vi "XPath String Sub-Parser_Tran.vi"(8 "error in (no error)":errorcluster, 10 "XPath expression":string, 11 "XML String":string) -> (0 "error out":errorcluster, 2 "Array of Results":string[](array[string]), 3 "XML String out":string)   [LabVIEW 2019]
doc: "Use an XPath expression to search an XML string. An array containing all instances matching the search criteria will be returned.\n\nFor more information on XPath: http://www.w3schools.com/xpath/xpath_intro.asp"
uses:
  <vilib>/xml/Close Reference(Node).vi
  <vilib>/xml/NI_XML.lvlib
  <resource>/objmgr/DOMUserDefRef.rc
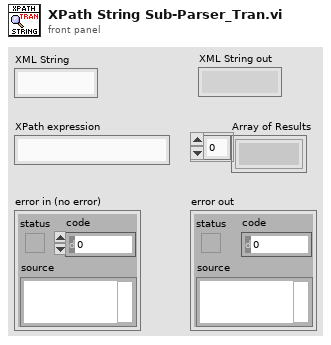
[diagram p1: front panel]
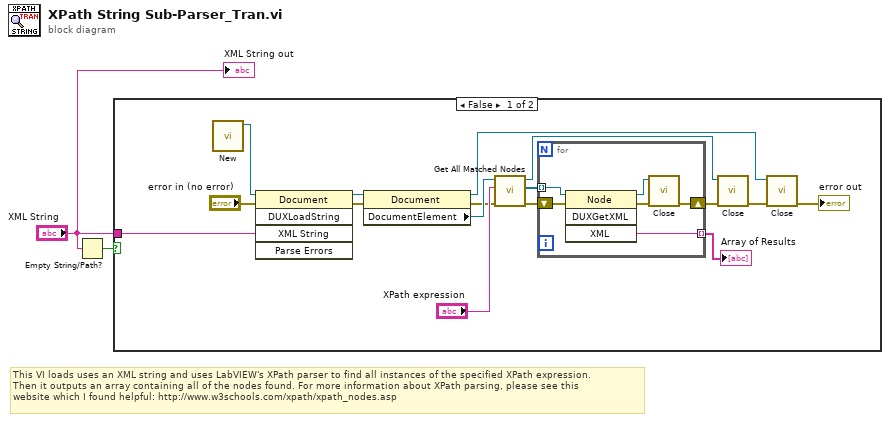
[diagram p0: block diagram]
diagram:
  # "This VI loads uses an XML string and uses LabVIEW's XPath parser to find all instances of the specified XPath expression. \nThen it outputs an array containing all of the nodes found. For more information about XPath parsing, please see this \nwebsite which I found helpful: http://www.w3schools.com/xpath/xpath_nodes.asp"
  n1 = Empty String/Path?(string/path="XML String") -> (empty?=w1:bool)
  n2 = case shown="False" w1 {
    tunnel: "XML String" -> [w4 _]
    frame False {
      n3 = call <vilib>:"New.vi"() -> ("DOM document out"=w18:refnum<k20>)  [unwired: 8 in, 1 out]
      n4 = invoke class="Document" method="DUXLoadString"(reference=w18, error in="error in (no error)", "XML String"=w4) -> (reference out=w16:refnum<k20>, error out=w15:errorcluster)  [unwired: 2 in, 3 out]
      n5 = property class="Document"(reference=w16, error in=w15) -> (reference out=w6:refnum<k20>, error out=w7:errorcluster, "DocumentElement"=w8:refnum<k20>)
      n6 = call <vilib>:"Get All Matched Nodes.vi"("error in (no error)"=w7, "XPath expression"="XPath expression", "node in"=w8) -> ("error out"=w12:errorcluster, "node result array"=w11:refnum<k20>[], "node out"=w5:refnum<k20>)  [unwired: 6 in]
      n7 = for {
        tunnel: w11 -> [w24] mode=indexing
        tunnel: [w23] -> w13 mode=indexing
        shift-right: [w19] -> w10
        shift-left: w12 -> [w22]
        n8 = invoke class="Node" method="DUXGetXML"(reference=w24, error in=w22) -> (reference out=w21:refnum<k20>, error out=w20:errorcluster, "XML"=w23:string)  [unwired: 2 in, 1 out]
        n9 = call-poly <vilib>:"Close.vi"("error in (no error)"=w20, "node"=w21) -> ("error out"=w19:errorcluster)  [unwired: 7 in]
      }
      "Array of Results" <- w13
      n10 = call-poly <vilib>:"Close.vi"("error in (no error)"=w10, "node"=w5) -> ("error out"=w9:errorcluster)  [unwired: 7 in]
      n11 = call-poly <vilib>:"Close.vi"("error in (no error)"=w9, "node"=w6) -> ("error out"=→"error out":errorcluster)  [unwired: 7 in]
    }
    frame True {
    }
  }
  "XML String out" <- "XML String"
